vi "SetUp.vi"(8 "error in (no error)":errorcluster, 11 "Prueba02 in":refnum<class "Prueba02.lvclass">) -> (0 "error out":errorcluster, 3 "Prueba02 out":refnum<class "Prueba02.lvclass">)   [LabVIEW 2019, in "Prueba02.lvclass"]
uses:
  Prueba02.lvclass
  Prueba02.lvclass/Prueba02.ctl
  Prueba/Prueba.lvclass
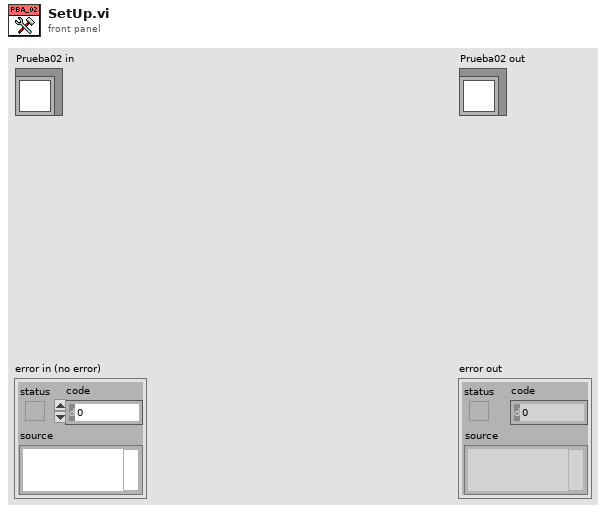
[diagram p1: front panel]
types:
  T1 = typedef "Prueba02.lvclass/BD.ctl" = cluster{"NivelMax_A":dbl, "NivelMax_C":dbl, "NivelMax_Z":dbl, "NivelMax_F":dbl, "Incertidumbres":dbl[]}
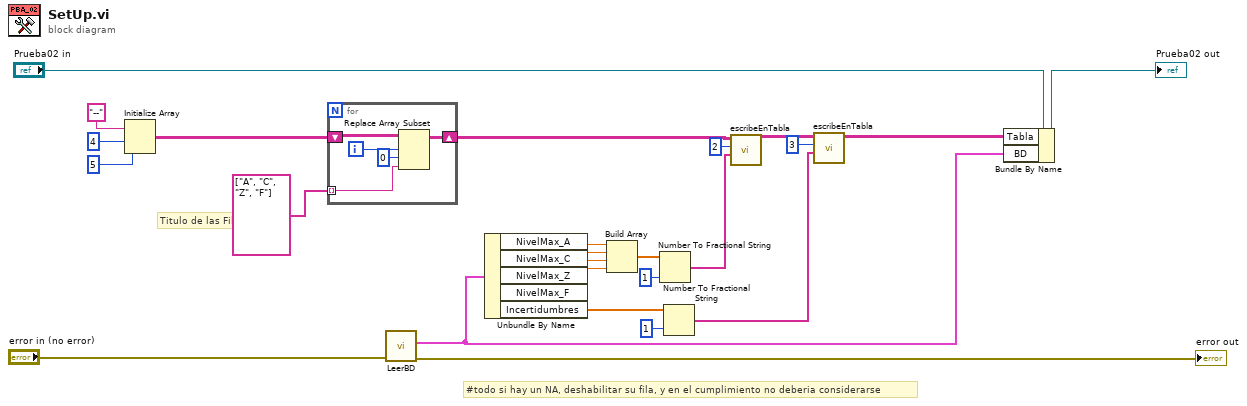
[diagram p0: block diagram]
diagram:
  # "#todo si hay un NA, deshabilitar su fila, y en el cumplimiento no deberia considerarse"
  # "Titulo de las Filas"
  n1 = Initialize Array("--", 4 ("dimension size"), 5 ("dimension size")) -> (w18:string[][])
  n2 = for {
    shift-right: [w29] -> w16
    shift-left: w18 -> [w30]
    tunnel: string[] ["A", "C", "Z", "F"] -> [w26] mode=indexing
    i -> [w28]
    n3 = Replace Array Subset(array=w30, new element=w26, index (row)=w28, index (col)=0 ("disabled index (col)")) -> (w29:string[][])
  }
  n4 = call "LeerBD.vi"("error in (no error)"="error in (no error)") -> ("error out"=→"error out":errorcluster, "BD"=w1:T1)  [unwired: 8 in, 1 out]
  n5 = Unbundle By Name(w1) -> ("NivelMax_A"=w15:dbl, "NivelMax_C"=w14:dbl, "NivelMax_Z"=w13:dbl, "NivelMax_F"=w12:dbl, "Incertidumbres"=w5:dbl[])
  n6 = Build Array(w15, w14, w13, w12) -> (w11:dbl[])
  n7 = Number To Fractional String(number=w11, precision (6)=i16 1) -> (F-format string=w9:string[])  [unwired: 2 in]
  n8 = Number To Fractional String(number=w5, precision (6)=i16 1) -> (F-format string=w4:string[])  [unwired: 2 in]
  n9 = call "escribeEnTabla.vi"("parametros"=w9, "col"=2, "tabla in"=w16) -> ("tabla out"=w3:string[][])  [unwired: 8 in]
  n10 = call "escribeEnTabla.vi"("parametros"=w4, "col"=3, "tabla in"=w3) -> ("tabla out"=w2:string[][])  [unwired: 8 in]
  n11 = Bundle By Name(cluster="Prueba02 in", "Tabla"=w2, "BD"=w1) -> (→"Prueba02 out":refnum<class "Prueba02.lvclass">)
